vi "ARCOSTranslate.vi"(7 "file (use dialog)":path, 8 "OP":enum16{"Export", "Import"}(ring), 11 "Front Panel":refnum<vi>) -> ()   [LabVIEW 2019]
panel:
  out "DataOut":T1(array[cluster])
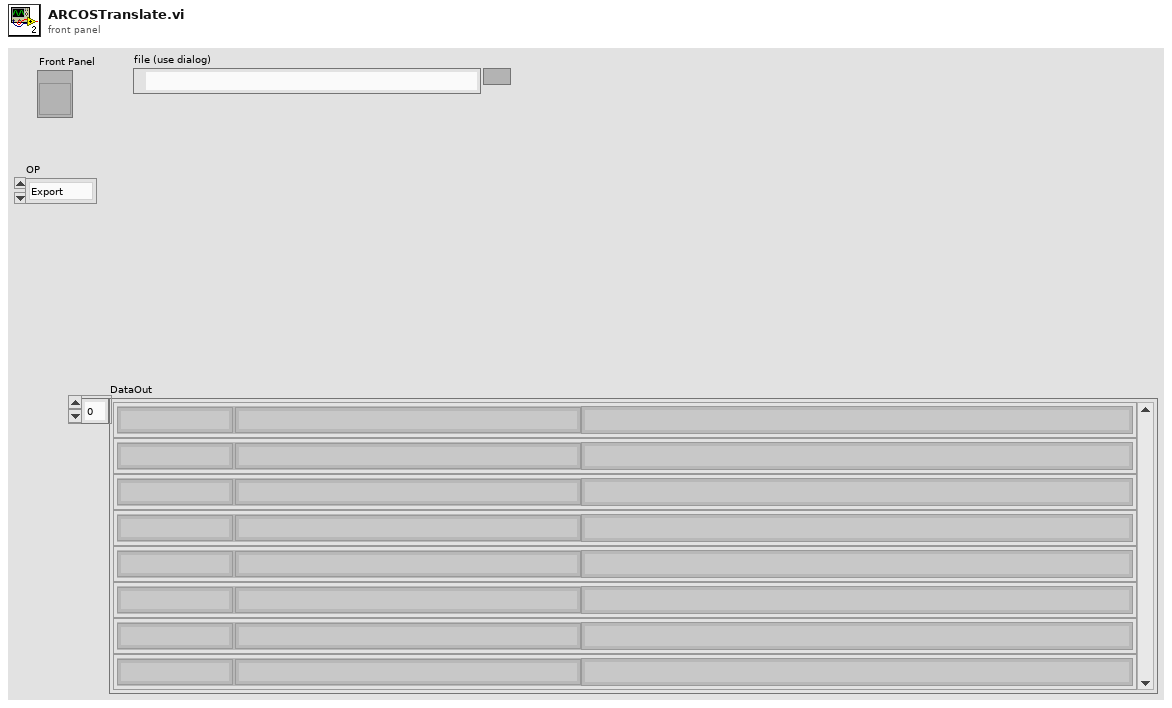
[diagram p1: front panel]
types:
  T1 = cluster{string, "Label":string, "Display":string}[]
  T2 = cluster{string, "Label.Text":string, "delimited string":string}[]
  T3 = cluster{"Type":string[], "Level":string[], "Data":string[]}
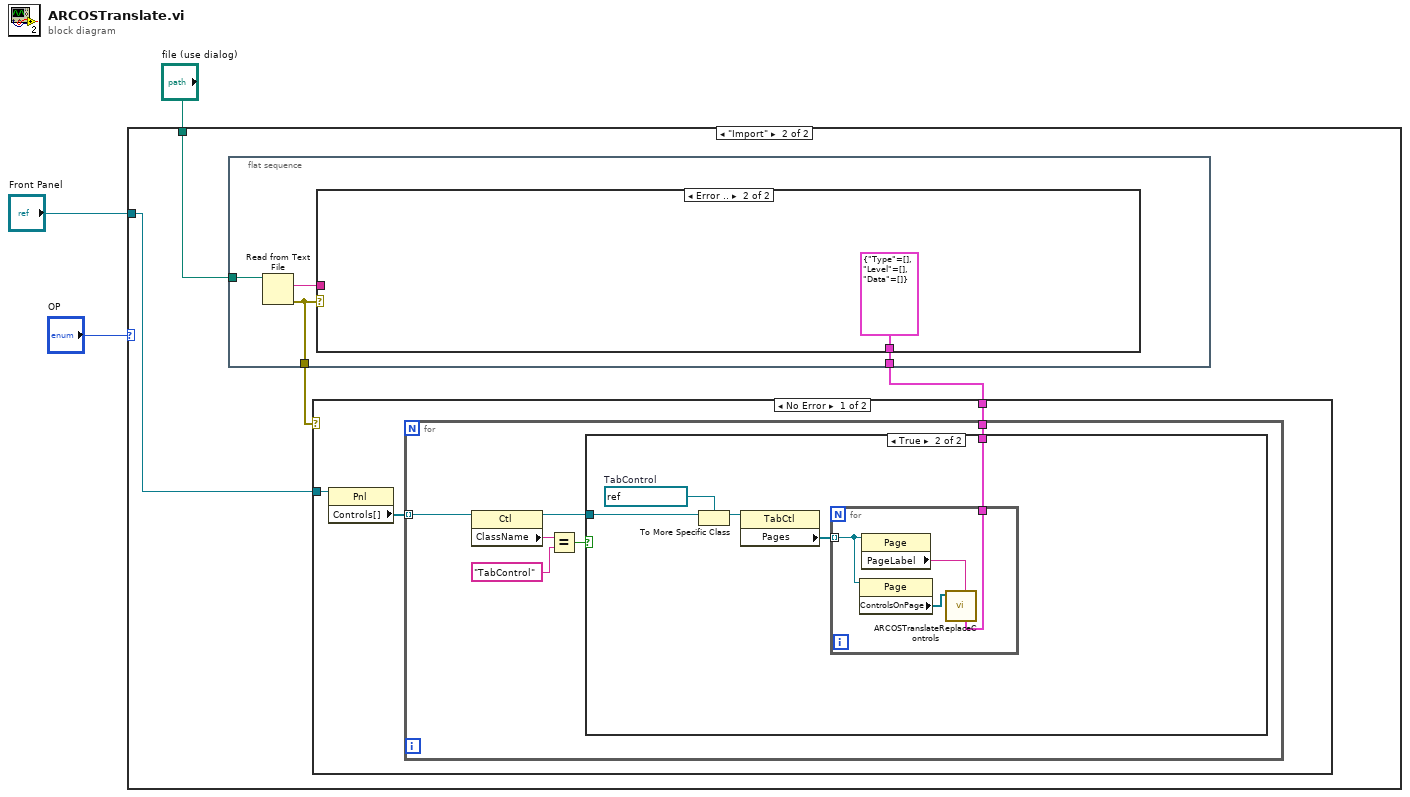
[diagram p0: block diagram]
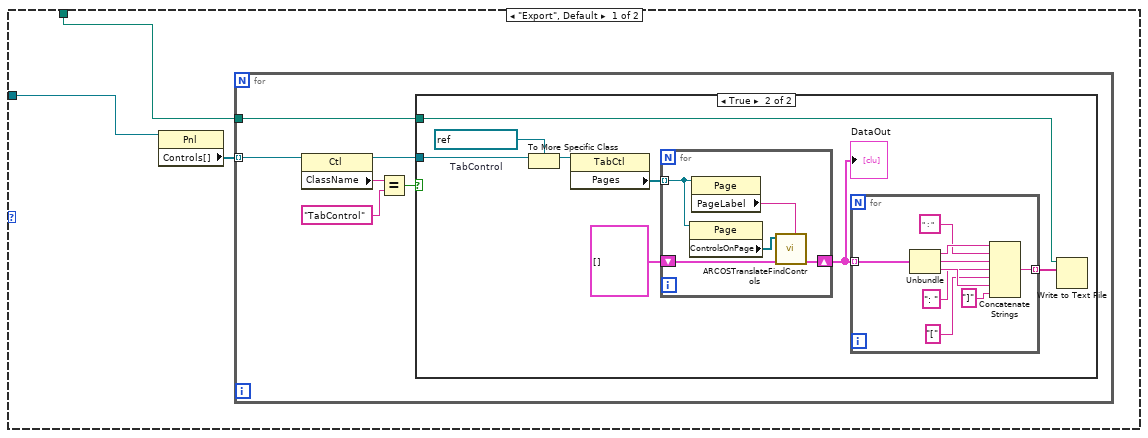
[diagram p2: hidden frame]
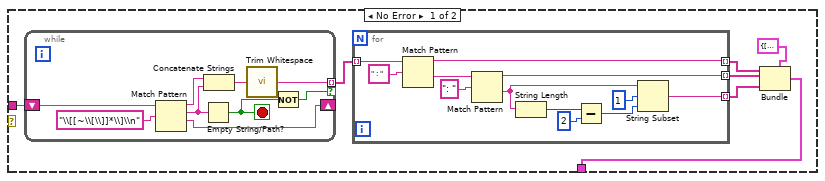
[diagram p6: hidden frame]
diagram:
  n1 = case shown="\"Import\"" "OP" {
    tunnel: "file (use dialog)" -> [w5 w38]
    tunnel: "Front Panel" -> [w4 w36]
    frame "Export", Default {
      n2 = property class="Pnl"(reference=w4) -> ("Controls[]"=w6:refnum<vi>[])  [unwired: 1 in, 2 out]
      n3 = for {
        tunnel: w6 -> [w12] mode=indexing
        tunnel: w5 -> [w7]
        n4 = property class="Ctl"(reference=w12) -> (reference out=w8:refnum<vi>, "ClassName"=w10:string)  [unwired: 1 in, 1 out]
        n5 = Equal?(x=w10, y="TabControl") -> (x = y?=w9:bool)
        n6 = case shown="True" w9 {
          tunnel: w8 -> [_ w20]
          tunnel: w7 -> [_ w13]
          frame False {
          }
          frame True {
            w19 = refnum<vi> refnum  # TabControl
            n7 = To More Specific Class(target class=w19, reference=w20) -> (specific class reference=w18:refnum<vi>)  [unwired: 1 in, 1 out]
            n8 = property class="TabCtl"(reference=w18) -> ("Pages"=w17:refnum<vi>[])  [unwired: 1 in, 2 out]
            n9 = for {
              tunnel: w17 -> [w31] mode=indexing
              shift-right: [w32] -> w15
              shift-left: T2 [] ("DataOut") -> [w33]
              n10 = property class="Page"(reference=w31) -> ("ControlsOnPage"=w34:refnum<vi>[])  [unwired: 1 in, 2 out]
              n11 = property class="Page"(reference=w31) -> ("PageLabel"=w30:string)  [unwired: 1 in, 2 out]
              n12 = call "ARCOSTranslateFindControls.vi"("Page Label"=w30, "DataIn"=w33, "ControlsOnPage"=w34) -> ("DataOut"=w32:T2)  [unwired: 8 in]
            }
            "DataOut" <- w15
            n13 = for {
              tunnel: w15 -> [w29] mode=indexing
              tunnel: [w26] -> w14 mode=indexing
              n14 = Unbundle(w29) -> (w28:string, "Label.Text"=w27:string, "delimited string"=w25:string)
              n15 = Concatenate Strings(w28, " : " ("string"), w27, ": ", "[" ("string"), w25, "]" ("string")) -> (w26:string)
            }
            n16 = Write to Text File(file (use dialog)=w13, text=w14) -> ()  [unwired: 2 in, 3 out]
          }
        }
      }
    }
    frame "Import" {
      n17 = flat-sequence {
        tunnel: w38 -> [w59]
        tunnel: [w58] -> w37
        tunnel: [w57] -> w35
        frame #0 {
          n18 = Read from Text File(file (use dialog)=w59) -> (text=w60:string, error out=w57:errorcluster)  [unwired: 3 in, 2 out]
          n19 = case shown="Error .." w57 {
            tunnel: w60 -> [w67 _]
            tunnel: [w62 T3 {"Type"=[], "Level"=[], "Data"=[]} ("cluster")] -> w58
            frame No Error {
              n20 = while {
                tunnel: [w83] -> w66 mode=indexing if=w80
                shift-right: [w84] -> _
                shift-left: w67 -> [w85]
                stop <- w81 stop-if-true
                n21 = Match Pattern(string=w85, regular expression="\\[[~\\[\\]]*\\]\\n") -> (before substring=w87:string, match substring=w86:string, after substring=w84:string)  [unwired: 1 in, 1 out]
                n22 = Empty String/Path?(string/path=w86) -> (empty?=w81:bool)
                n23 = Concatenate Strings(w87, w86) -> (w82:string)
                n24 = call <vilib>:"Trim Whitespace.vi"("string"=w82) -> ("trimmed string"=w83:string)  [unwired: 1 in]
                n25 = Not(x=w81) -> (.not. x?=w80:bool)
              }
              n26 = for {
                tunnel: w66 -> [w79] mode=indexing
                tunnel: [w70] -> w65 mode=indexing
                tunnel: [w69] -> w64 mode=indexing
                tunnel: [w68] -> w63 mode=indexing
                n27 = Match Pattern(string=w79, regular expression=" : ") -> (before substring=w70:string, after substring=w77:string)  [unwired: 1 in, 2 out]
                n28 = Match Pattern(string=w77, regular expression=": ") -> (before substring=w69:string, after substring=w74:string)  [unwired: 1 in, 2 out]
                n29 = String Length(string=w74) -> (length=w73:i32)
                n30 = Subtract(x=w73, y=2) -> (x-y=w71:i32)
                n31 = String Subset(string=w74, offset (0)=1, length (rest)=w71) -> (substring=w68:string)
              }
              n32 = Bundle(cluster=T3 {"Type"=[], "Level"=[], "Data"=[]}, "Type"=w65, "Level"=w64, "Data"=w63) -> (w62:T3)
            }
            frame Error {
            }
          }
        }
      }
      n33 = case shown="No Error" w35 {
        tunnel: w37 -> [w40 _]
        tunnel: w36 -> [w39 _]
        frame No Error {
          n34 = property class="Pnl"(reference=w39) -> ("Controls[]"=w41:refnum<vi>[])  [unwired: 1 in, 2 out]
          n35 = for {
            tunnel: w41 -> [w47] mode=indexing
            tunnel: w40 -> [w42]
            n36 = property class="Ctl"(reference=w47) -> (reference out=w43:refnum<vi>, "ClassName"=w45:string)  [unwired: 1 in, 1 out]
            n37 = Equal?(x=w45, y="TabControl") -> (x = y?=w44:bool)
            n38 = case shown="True" w44 {
              tunnel: w43 -> [_ w52]
              tunnel: w42 -> [_ w48]
              frame False {
              }
              frame True {
                w51 = refnum<vi> refnum  # TabControl
                n39 = To More Specific Class(target class=w51, reference=w52) -> (specific class reference=w50:refnum<vi>)  [unwired: 1 in, 1 out]
                n40 = property class="TabCtl"(reference=w50) -> ("Pages"=w49:refnum<vi>[])  [unwired: 1 in, 2 out]
                n41 = for {
                  tunnel: w49 -> [w55] mode=indexing
                  tunnel: w48 -> [w53]
                  n42 = property class="Page"(reference=w55) -> ("ControlsOnPage"=w56:refnum<vi>[])  [unwired: 1 in, 2 out]
                  n43 = property class="Page"(reference=w55) -> ("PageLabel"=w54:string)  [unwired: 1 in, 2 out]
                  n44 = call "ARCOSTranslateReplaceControls.vi"("TranslateData"=w53, "Page Label"=w54, "ControlsOnPage"=w56) -> ()  [unwired: 9 in]
                }
              }
            }
          }
        }
        frame Error {
        }
      }
    }
  }
